vi "GV N pixelclock per line.vi"() -> ()   [LabVIEW 2017]
panel:
  out "NpixelclockPerLine":i16
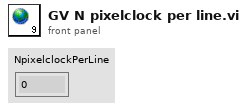
[diagram p1: front panel]
diagram:
